vi "Add Unique Child.vi"(8 "error in":errorcluster, 9 "Child":string, 10 "Parent":string, 11 "Tree Refnum in":refnum<vi>) -> (0 "error out":errorcluster, 3 "Tree Refnum out":refnum<vi>)   [LabVIEW 2019, in "Configuration.lvlib" / "Configuration.lvclass"]
uses:
  Configuration.lvclass
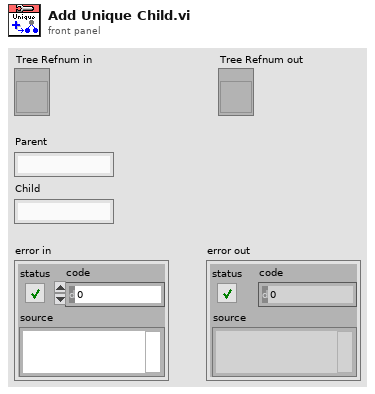
[diagram p1: front panel]
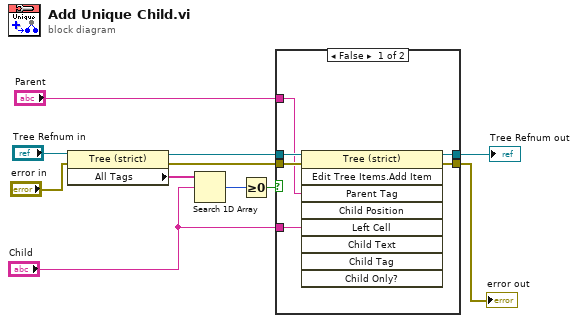
[diagram p0: block diagram]
diagram:
  n1 = property class="Tree (strict)"(reference="Tree Refnum in", error in="error in") -> (reference out=w10:refnum<vi>, error out=w4:errorcluster, "All Tags"=w8:string[])
  n2 = Search 1D Array(1D array=w8, element="Child") -> (index of element=w7:i32)  [unwired: 1 in]
  n3 = Greater Or Equal To 0?(x=w7) -> (x >= 0?=w6:bool)
  n4 = case shown="False" w6 {
    tunnel: w10 -> [w17 w19]
    tunnel: [w16 w19] -> w9
    tunnel: "Child" -> [w15 _]
    tunnel: w4 -> [w14 w18]
    tunnel: [w13 w18] -> w3
    tunnel: "Parent" -> [w12 _]
    frame False {
      n5 = invoke class="Tree (strict)" method="Edit Tree Items.Add Item"(reference=w17, error in=w14, "Parent Tag"=w12, "Left Cell"=w15) -> (reference out=w16:refnum<vi>, error out=w13:errorcluster)  [unwired: 5 in, 7 out]
    }
    frame True {
    }
  }
  "error out" <- w3
  "Tree Refnum out" <- w9
